vi "Read from EEPROM.vi"(8 "error in (no error)":errorcluster, 10 "EEPROM Index":u8, 11 "VISA resource name":refnum<visa-resource-name>) -> (0 "error out":errorcluster, 2 "ASCII Data":string, 3 "VISA resource name out":refnum<visa-resource-name>)   [LabVIEW 2012, in "Ocean Optics 2000 4000.lvlib"]
doc: "Reads data saved in the EEPROM based on the address entered."
uses:
  Ocean Optics 2000 4000.lvlib
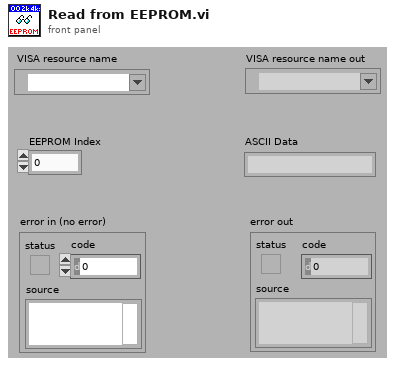
[diagram p1: front panel]
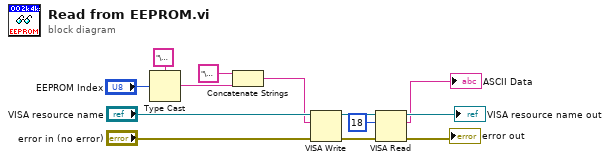
[diagram p0: block diagram]
diagram:
  n1 = Type Cast(type="\u0000", x="EEPROM Index") -> (*(type *) &x=w9:string)
  n2 = Concatenate Strings("\u0005" ("string"), w9) -> (w7:string)
  n3 = VISA Write(VISA resource name="VISA resource name", write buffer=w7, error in (no error)="error in (no error)") -> (VISA resource name out=w5:refnum<visa-resource-name>, error out=w6:errorcluster)  [unwired: 1 out]
  n4 = VISA Read(VISA resource name=w5, byte count=u32 18, error in (no error)=w6) -> (VISA resource name out=→"VISA resource name out":refnum<visa-resource-name>, read buffer=→"ASCII Data":string, error out=→"error out":errorcluster)  [unwired: 1 out]
